vi "ILYA_ADQ_GetData_Default.vi"(5 "buffer_chB_in":i16[](array[numeric]), 7 "buffer_chA_in":i16[](array[numeric]), 8 "error in":errorcluster, 10 "samples_per_record":u32, 11 "adq_cu_ptr":u32) -> (0 "error out":errorcluster, 3 "adq_cu_ptr":u32, 4 "buffer_chB_out":i16[](array[numeric]), 6 "buffer_chA_out":i16[](array[numeric]))   [LabVIEW 2013]
uses:
  GetData_DLL.dll
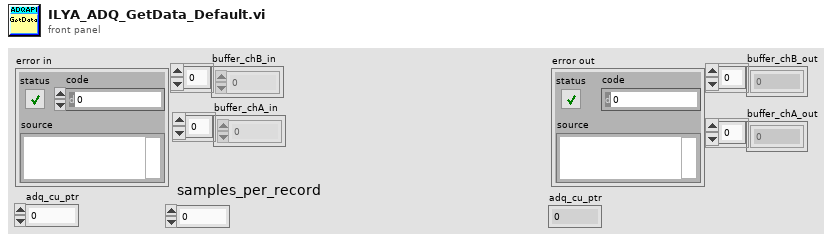
[diagram p1: front panel]
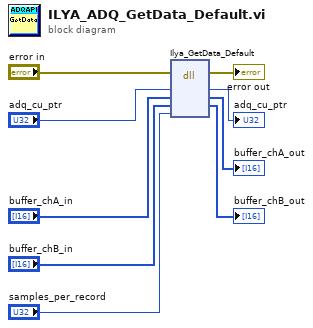
[diagram p0: block diagram]
diagram:
  n1 = dll-call lib="C:/Users/astafiev/Desktop/IlyaDrive/@photonCounting/LabView_Imperium/GetData_DLL.dll" fn="Ilya_GetData_Default"(error in="error in", "adq_cu_ptr"="adq_cu_ptr", "buffer_chA"="buffer_chA_in", "buffer_chB"="buffer_chB_in", "samples_per_record"="samples_per_record") -> (error out=→"error out":errorcluster, "adq_cu_ptr"=→"adq_cu_ptr":u32, "buffer_chA"=→"buffer_chA_out":i16[], "buffer_chB"=→"buffer_chB_out":i16[])  [unwired: 4 in, 1 out]
